vi "DTC.vi"(0 "System no.":i32=1 min=1 max=4 step=1, 2 "DDL table":string[](array[string]), 3 "All tables?":bool, 5 "error in":errorcluster) -> (19 "error out":errorcluster)   [LabVIEW 2020]
doc: "Clears DDL table.\n\nE-710: All tables? must be FALSE.\nE-712: All tables? must be FALSE.\nE-725, E-727: All tables? must be FALSE.\nE-753, E-754: All tables? must be FALSE.\nE-761: All tables? must be FALSE."
panel:
  # "Clears DDL table."
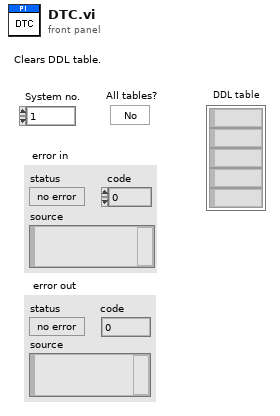
[diagram p1: front panel]
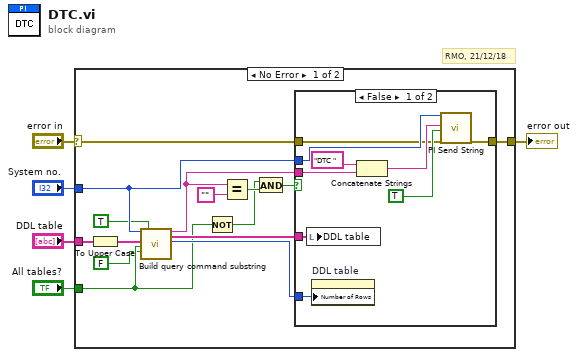
[diagram p0: block diagram]
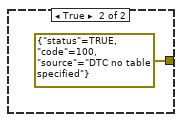
[diagram p2: hidden frame]
diagram:
  # "RMO, 21/12/18"
  n1 = case shown="No Error" "error in" {
    selector: "error in" -> [w8 w31]
    tunnel: "DDL table" -> [w20 _]
    tunnel: "System no." -> [w17 _]
    tunnel: "All tables?" -> [w13 _]
    tunnel: [w6 w31] -> w2
    frame No Error {
      n2 = To Upper Case(1:w20) -> (0:w11:string[])
      n3 = call "Build query command substring.vi"("System no."=w17, "Axes to query in"=w11, "Query\nAll axes?"=w13, "For all axes: use\nAxis identifier?"=FALSE ("For all axes: use\nAxis identifier?"), "With space?"=TRUE) -> ("Command substring"=w18:string, "Axes to query out"=w16:string[], "Number of rows"=w15:u32)  [unwired: 1 in, 11 out]
      n4 = Not(x=w13) -> (.not. x?=w12:bool)
      n5 = Equal?(x=w18, y="" ("x")) -> (x = y?=w14:bool)
      n6 = And(x=w12, y=w14) -> (x .and. y?=w7:bool)
      n7 = case shown="False" w7 {
        tunnel: w18 -> [w26 _]
        tunnel: w17 -> [w25 _]
        tunnel: w16 -> [w24 _]
        tunnel: w15 -> [w23 _]
        tunnel: w8 -> [w22 _]
        tunnel: [w21 errorcluster {"status"=TRUE, "code"=100, "source"="DTC no table specified"} ("error out")] -> w6
        frame False {
          n8 = local write "DDL table"(w24) -> ()
          n9 = property on="DDL table" class="Arr (strict)"("Number of Rows"=w23) -> ()  [unwired: 2 in, 2 out]
          n10 = Concatenate Strings("DTC ", w26) -> (w27:string)
          n11 = call "PI Send String.vi"("System no."=w25, "String to send"=w27, "Attach termination char.?"=TRUE ("Attach Linefeed?"), "error in"=w22) -> ("error out"=w21:errorcluster)  [unwired: 15 out]
        }
        frame True {
        }
      }
    }
    frame Error {
    }
  }
  "error out" <- w2
